vi "SwissSPAD2 Live.vi"() -> ()   [LabVIEW 2019]
uses:
  SS2 Live Internal Variables.ctl
  <vilib>/vision/Image Controls.llb/IMAQ Image.ctl
  SS2 Live_Image ROI Information.ctl
  Phasor/Image Binning Options.ctl
  SS2 Q [Element].ctl
  SS2 Q Event List.ctl
  Sound/System Sounds List.ctl
  SS2 Live_Settings List.ctl
  Image/Image Display to Clipboard Options.ctl
  Image/Image Display Palette Information.ctl
  Image/Image Display Palette Type.ctl
  SS2 Live_Internal Data List.ctl
  SS2 Live_Windows List.ctl
  SS2 Live_Globals.vi
  C:/UCLA Thinkpad Google Drive/LabVIEW 2019 SP1/builds/SS2 Live Distribution/Opal Kelly/C# Wrapper/libFrontPanel-csharp.dll
  Opal Kelly/C# Wrapper/libFrontPanel-csharp.dll
  Variant/Variant to Data/Variant to Data.lvlib
  Notebook/Notebook.lvlib
  Rich Text Box/Rich Text Box.lvlib
panel:
  out "Image":T1(plugin-control)
  out "Saving in progress":bool
  out "Progress":u8(slide) scale=0.0..100.0
  in  "Record":bool
  in  "Animated Busy Icon":bool=TRUE
  out "Message":string
  in  "Live":bool
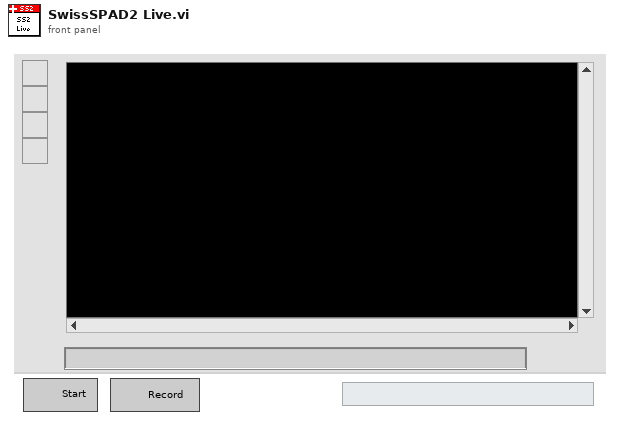
[diagram p1: front panel]
types:
  T1 = typedef "IMAQ Image.ctl" = refnum<image>
  T2 = typedef "SS2 Q [Element].ctl" = cluster{"SS2 Q Event":T3, "Data":variant}
  T3 = typedef "SS2 Q Event List.ctl" = enum16{"---- UI ----", "Idle", "Initialization", "Quit", "---- DAQ ----", "Start Recording", "Start Live Acquisition", "Initialize Recording Mode", "Initialize FPGA (Live Mode)", "Get Image Set", "Get Single Image", "Update Image Display", "Stop Live Acquisition", "Stop Data Recording", "---- Image ----", "Copy Data to Clipboard", "Set Image Palette", "Save Displayed Image with Overlay", "Save Image Data as TIFF"}
  T4 = typedef "SS2 Live Internal Variables.ctl" = cluster{"okCFrontPanelDevices Refnum":refnum<k24>, "Device Refnum":refnum<k24>, "Display Image":T1, "# Live Images":i32, "relative s":dbl, "# Image Sets":i32, "Message":string, "Current Image Set":i32, "# Datasets":i32, "Current Dataset":i32, "Live Mode":bool, "Recording Mode":bool, "Record Button":refnum<vi>, "Live Button":refnum<vi>, "SS2 Live Gate Data Q Name":string, "Discard First Image":bool, "Image Information":T5, "Image Binning Options":T6}
  T5 = typedef "SS2 Live_Image ROI Information.ctl" = cluster{"Save ROI Only":bool, "Left":u16, "Top":u16, "Right":u16, "Bottom":u16, "Use Current ROI":bool}
  T6 = typedef "Image Binning Options.ctl" = cluster{"Use Image Binning":bool, "X Bin":i32, "Y Bin":i32}
  T7 = typedef "SS2 Live_Settings List.ctl" = enum16{"FPGA:Bitfile Path", "FPGA:Bitfile Version", "Acquisition Parameters:SS2 DAQ Parameters", "Acquisition Parameters:Gate Configuration Array", "Acquisition Parameters:Buffer Size (# Gates)", "File Information:File Information", "File Information:# Datasets in Series", "Image Parameters:Image ROI Information", "Image Parameters:Image Binning Options", "UI Parameters:Histogram Bins Number"}
  T8 = typedef "System Sounds List.ctl" = enum16{"Alarm01", "Alarm02", "Alarm03", "Alarm04", "Alarm05", "Alarm06", "Alarm07", "Alarm08", "Alarm09", "Alarm10", "chimes", "chord", "ding", "notify", "recycle", "Ring01", "Ring02", "Ring03", "Ring04", "Ring05", "Ring06", "Ring07", "Ring08", "Ring09", "Ring10", "ringout", "Speech Off", "Speech On", "Speech Sleep", "tada", "Windows Background", "Windows Balloon", "Windows Battery Critical", "Windows Battery Low", "Windows Critical Stop", "Windows Default", "Windows Ding", "Windows Error", "Windows Exclamation", "Windows Feed Discovered", "Windows Foreground", "Windows Hardware Fail", "Windows Hardware Insert", "Windows Hardware Remove", "Windows Information Bar", "Windows Logoff Sound", "Windows Logon", "Windows Menu Command", "Windows Message Nudge", "Windows Minimize", "Windows Navigation Start", "Windows Notify Calendar", "Windows Notify Email", "Windows Notify Messaging", "Windows Notify System Generic", "Windows Notify", "Windows Pop-up Blocked", "Windows Print complete", "Windows Proximity Connection", "Windows Proximity Notification", "Windows Recycle", "Windows Restore", "Windows Ringin", "Windows Ringout", "Windows Shutdown", "Windows Startup", "Windows Unlock", "Windows User Account Control"}
  T9 = typedef "Image Display to Clipboard Options.ctl" = cluster{"Include Overlay (T)":bool, "Image Only (T)":bool}
  T10 = cluster{"CtlRef":refnum<vi>, "Image to Clipboard Options":T9}
  T11 = typedef "Image Display Palette Information.ctl" = cluster{"Palette Name [# Colors,int?,inv?]":string, "Palette Type":T12, "Palette Colors":u32[], "Interpolate?":bool}
  T12 = typedef "Image Display Palette Type.ctl" = u32
  T13 = typedef "Rich Text Box.lvlib/Text Formatting.ctl" = cluster{"Font":string, "Text Color":T14, "Text Background Color":T14, "Text Style":enum16{"Regular", "Bold", "Italic", "Underline", "Strikeout"}, "Font Size (Points)":dbl, "Text Alignment":i32}
  T14 = typedef "Rich Text Box.lvlib/Text Colors.ctl" = enum16{"Unchanged", "Black", "Blue", "Gray", "Green", "Red", "White"}
  T15 = typedef "Save File Format.ctl" = enum16{"PNG", "JPEG", "BMP"}
  T16 = typedef "SS2 Live_Internal Data List.ctl" = enum16{"Number of pending file saving tasks", "File Saving Tasks Information", "Current Image ROI Information"}
  T17 = typedef "SS2 Live_Windows List.ctl" = enum16{"Settings Window", "Notebook Window", "Histogram Window", "About Window", "SS2 Live Window"}
  T18 = cluster{"Global Rectangle":i32[], "Contours":cluster{"Contour Type":u32, "ROI Type":u32, "Points":i32[]}[]}
  T19 = typedef "SS2 Live_File Saving Task Information.ctl" = cluster{"File Path":string, "# Saved Images":i32, "# Images (Total)":i32, "File Size (Bytes)":i64}
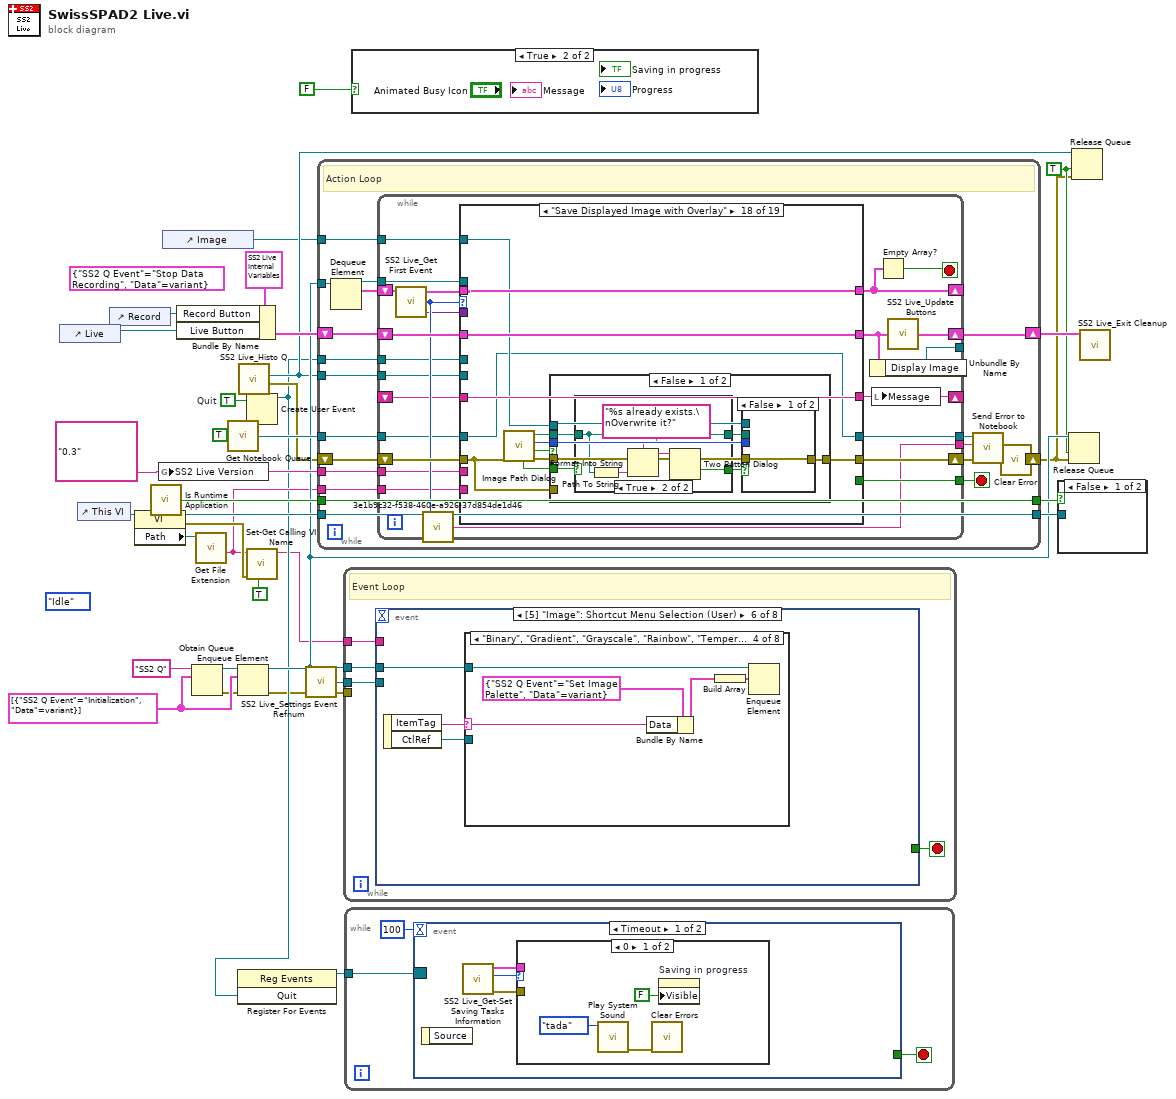
[diagram p0: block diagram]
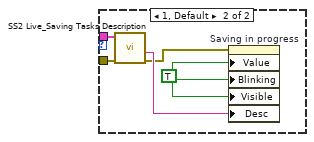
[diagram p2: hidden frame]
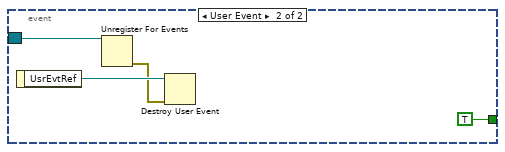
[diagram p3: hidden frame]
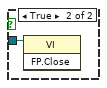
[diagram p5: hidden frame]
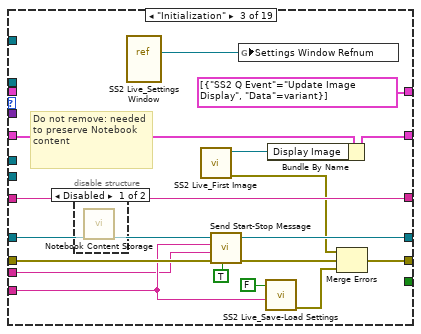
[diagram p8: hidden frame]
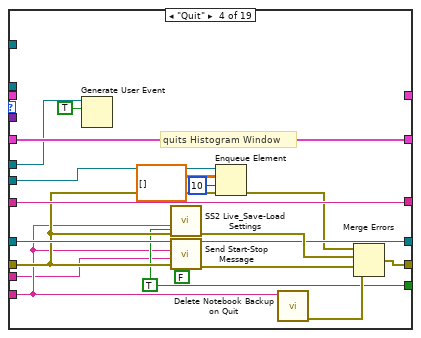
[diagram p10: hidden frame]
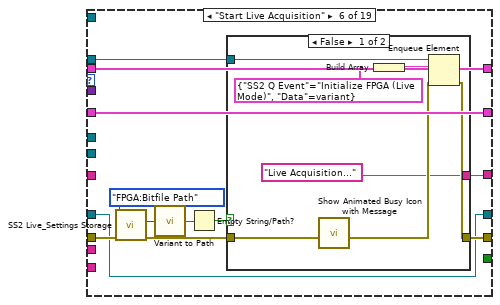
[diagram p12: hidden frame]
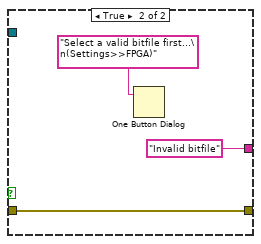
[diagram p13: hidden frame]
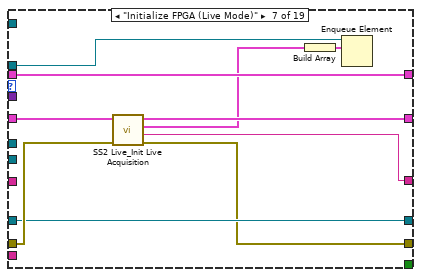
[diagram p14: hidden frame]
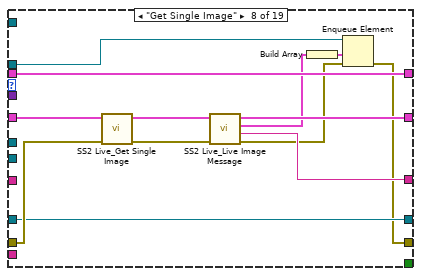
[diagram p15: hidden frame]
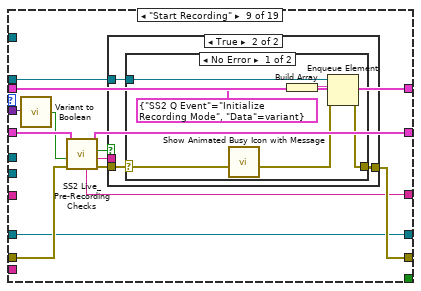
[diagram p16: hidden frame]
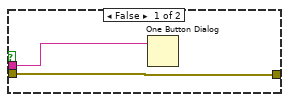
[diagram p17: hidden frame]
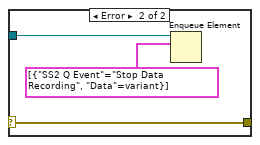
[diagram p18: hidden frame]
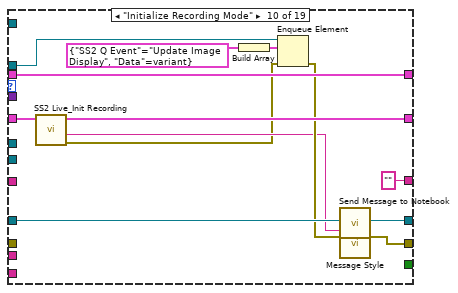
[diagram p19: hidden frame]
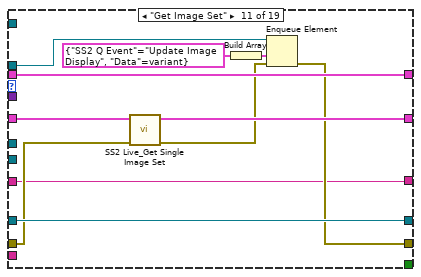
[diagram p20: hidden frame]
diagram:
  w9 = TRUE  # Quit
  (unwired) T2 {"SS2 Q Event"=enum."Stop Data Recording", "Data"=variant} ("f")
  w15 = TRUE ("force destroy? (F)")
  w18 = T2[] [{"SS2 Q Event"=enum."Initialization", "Data"=variant}] ("element")
  (unwired) SS2_Q_Event_List."Idle" ("SS2 Q Event")
  w20 = "0.3" ("SS2 Live Version")
  n1 = control-ref of="Live"() -> (w11:refnum<vi>)
  n2 = control-ref of="This VI"() -> (w32:refnum<vi>)
  n3 = control-ref of="Record"() -> (w10:refnum<vi>)
  n4 = property class="VI"(reference=w32) -> (reference out=w29:refnum<vi>, error out=w28:errorcluster, "Path"=w16:path)  [unwired: 1 in]
  n5 = call "Is Runtime Application.vi"() -> ("Runtime ?"=w34:bool)  [unwired: 8 in, 1 out]
  n6 = global write "SS2 Live_Globals.vi" "SS2 Live Version"(w20) -> ()
  n7 = control-ref of="Image"() -> (w1:refnum<vi>)
  n8 = Bundle By Name(cluster=T4 {"okCFrontPanelDevices Refnum"=refnum, "Device Refnum"=refnum, "Display Image"=refnum, "# Live Images"=0, "relative s"=nan, "# Image Sets"=0, "Message"="", "Current Image Set"=0, "# Datasets"=0, "Current Dataset"=0, "Live Mode"=FALSE, "Recording Mode"=FALSE, "Record Button"=refnum, "Live Button"=refnum, "SS2 Live Gate Data Q Name"="SS2 Live Gate Data Q", "Discard First Image"=FALSE, "Image Information"={"Save ROI Only"=FALSE, "Left"=0, "Top"=0, "Right"=0, "Bottom"=0, "Use Current ROI"=FALSE}, "Image Binning Options"={"Use Image Binning"=FALSE, "X Bin"=1, "Y Bin"=1}}, "Record Button"=w10, "Live Button"=w11) -> (w25:T4)
  n9 = Obtain Queue(name (unnamed)="SS2 Q", element data type=w18) -> (queue out=w21:refnum<queue>, error out=w5:errorcluster)  [unwired: 3 in, 1 out]
  n10 = call <vilib>:"Get File Extension.vi"("file"=w16) -> ("filename without extension"=w17:string)  [unwired: 6 in, 4 out]
  n11 = call "Get Notebook Queue.vi"("create if not found? (T)"=TRUE ("create if not found? (F)")) -> ("Notebook Queue"=w22:refnum<queue>)  [unwired: 8 in]
  n12 = Enqueue Element(queue=w21, element=w18, error in (no error)=w5) -> (queue out=w19:refnum<queue>, error out=w6:errorcluster)  [unwired: 1 in, 1 out]
  n13 = call "SS2 Live_Histo Q.vi"() -> ("error out"=w13:errorcluster, "SS2 Live Histo Q"=w12:refnum<queue>)  [unwired: 6 in]
  n14 = Create User Event(user event datatype=w9) -> (user event=w7:refnum<user-event>)  [unwired: 1 in, 1 out]
  n15 = register-events(w7) -> (reference out=w8:refnum<event-registration>)  [unwired: 2 in, 1 out]
  n16 = call "Set-Get Calling VI Name.vi"("Set/Get (F)"=TRUE, "Error In"=w28, "Calling VI Name"=w17) -> ("Calling VI Name"=w2:string)  [unwired: 7 in, 1 out]
  n17 = call "SS2 Live_Settings Event Refnum.vi"("Error In"=w6) -> ("Settings Event Refnum"=w3:refnum<user-event>, "Error Out"=w4:errorcluster)  [unwired: 7 in]
  n18 = while {
    tunnel: w19 -> [w55]
    tunnel: w34 -> [w50]
    tunnel: [w50] -> w33
    tunnel: w29 -> [w49]
    tunnel: [w49] -> w31
    shift-right: [w42] -> w14
    shift-left: w13 -> [w52]
    shift-right: [w47] -> w24
    shift-left: w25 -> [w48]
    tunnel: w22 -> [w46]
    tunnel: w20 -> [w40]
    tunnel: w17 -> [w39]
    tunnel: w12 -> [w38]
    tunnel: w7 -> [w37]
    tunnel: w1 -> [w36]
    stop <- w53 stop-if-true
    # "Action Loop"
    n19 = Dequeue Element(queue=w55) -> (queue out=w51:refnum<queue>, element=w54:T2[])  [unwired: 2 in, 2 out]
    n20 = while {
      tunnel: [w79] -> w53
      tunnel: w51 -> [w77]
      shift-right: [w76] -> w45
      shift-left: w52 -> [w78]
      shift-right: [w73] -> _
      shift-left: w54 -> [w75]
      shift-right: [w60] -> w47
      shift-left: w48 -> [w71]
      tunnel: w46 -> [w68]
      tunnel: [w65] -> w44
      tunnel: [w69] -> w41
      tunnel: w40 -> [w67]
      tunnel: w39 -> [w66]
      shift-right: [w64] -> _
      shift-left: _ -> [w63]
      tunnel: w38 -> [w61]
      tunnel: w37 -> [w59]
      tunnel: [w57] -> _
      tunnel: w36 -> [w56]
      stop <- w72 stop-if-true
      n21 = call "SS2 Live_Get First Event.vi"("SS2 Q Element"=w75) -> ("Data"=w62:variant, "SS2 Q Event"=w70:T3, "SS2 Q Elements"=w74:T2[])  [unwired: 2 in]
      n22 = call "3e1b9c32-f538-460e-a926-37d854de1d46.vi"("Enum"=w70) -> ("String"=w69:string)
      n23 = case shown="\"Save Displayed Image with Overlay\"" w70 {
        tunnel: [_ _ _ w113 _ _ _ _ _ _ _ _ _ _ _ _ _ _ _] -> w79
        tunnel: w78 -> [w84 w89 w98 w114 w128 w133 w157 w169 w182 _ w221 w228 w240 w257 w275 w283 w288 w305 w342]
        tunnel: w77 -> [_ _ _ _ _ w140 w160 w173 w186 w213 w224 w234 w246 w270 _ _ _ _ _]
        tunnel: [w84 w89 w104 w123 w128 w139 w151 w161 w185 w204 w215 w237 w244 w263 w275 w277 w289 w310 w342] -> w76
        tunnel: w74 -> [w83 w88 _ _ w127 w137 w158 w171 w184 w211 w223 w236 _ _ w274 w287 w302 w314 w341]
        tunnel: [w83 w88 T2[] [{"SS2 Q Event"=enum."Update Image Display", "Data"=variant}] ("SS2 Q Elements") _ w127 w137 w158 w171 w184 w211 w223 w236 _ _ w274 w287 w302 w314 w341] -> w73
        tunnel: w71 -> [w80 w87 w105 w121 w124 w136 w156 w170 w177 w208 w220 w232 w241 w251 w271 w282 w293 w313 w340]
        tunnel: [w80 w87 w92 w121 w124 w136 w154 w166 w176 w207 w217 w230 w239 w268 w271 w282 w293 w313 w340] -> w58
        tunnel: w61 -> [_ _ _ w117 _ _ _ _ _ _ _ _ _ _ _ _ _ _ _]
        tunnel: w68 -> [w82 w86 w100 w115 w126 w130 w155 w167 w181 w206 w222 w235 w243 w265 w273 w286 w301 w303 w339]
        tunnel: w67 -> [_ _ w96 w109 _ _ _ _ _ _ _ _ _ _ _ _ _ _ _]
        tunnel: w66 -> [_ _ w97 w110 _ _ _ _ _ _ _ _ _ _ _ _ _ _ _]
        tunnel: [w82 w86 w100 w115 w126 w130 w155 w167 w181 w206 w222 w235 w243 w265 w273 w286 w301 w303 w339] -> w65
        tunnel: [w81 w85 w102 w120 w125 w129 w152 w163 w179 "" ("Message") w214 w226 "Live Mode stopped" ("Message") w262 w272 w285 w300 w312 w338] -> w64
        tunnel: w63 -> [w81 w85 w102 w120 w125 _ _ _ _ _ w214 w225 _ _ w272 w285 w300 w312 w338]
        tunnel: w62 -> [_ _ _ _ _ _ _ _ w175 _ _ _ _ _ _ w284 w295 _ _]
        tunnel: w59 -> [_ _ _ w108 _ _ _ _ _ _ _ _ _ _ _ _ _ _ _]
        tunnel: w56 -> [_ _ _ _ _ _ _ _ _ _ _ _ _ _ _ _ w290 w311 _]
        frame "---- UI ----" {
        }
        frame "Idle", Default {
        }
        frame "Initialization" {
          # "Do not remove: needed to preserve Notebook content"
          n24 = disable-structure shown="Disabled" {
            frame Disabled {
              n25 = call "Notebook Content Storage.vi"() -> ()  [unwired: 10 in, 2 out]
            }
            frame Enabled {
            }
          }
          n26 = vi-ref "SS2 Live_Settings Window.vi"() -> (w101:refnum<vi>)
          n27 = call "SS2 Live_First Image.vi"() -> ("error out"=w90:errorcluster, "Image"=w91:T1)  [unwired: 10 in]
          n28 = call "Send Start-Stop Message.vi"("Start(T)/Stop(F)"=TRUE ("Start(F)/Stop(T)"), "Error In"=w98, "Version number"=w96, "Software Name"=w97, "Notebook Queue"=w100) -> ("Error Out"=w99:errorcluster)  [unwired: 6 in]
          n29 = global write "SS2 Live_Globals.vi" "Settings Window Refnum"(w101) -> ()
          n30 = call "SS2 Live_Save-Load Settings.vi"("Load(F)/Save (T)"=FALSE, "App Name"=w97) -> ("Error Out"=w103:errorcluster)  [unwired: 8 in, 1 out]
          n31 = Bundle By Name(cluster=w105, "Display Image"=w91) -> (w92:T4)
          n32 = Merge Errors(w90, w99, w103) -> (w104:errorcluster)
        }
        frame "Quit" {
          w113 = TRUE
          # "quits Histogram Window"
          n33 = Generate User Event(user event=w108, event data cluster=TRUE ("event data")) -> ()  [unwired: 2 in, 2 out]
          n34 = call "SS2 Live_Save-Load Settings.vi"("Load(F)/Save (T)"=w113, "Error In"=w114, "App Name"=w110) -> ("Error Out"=w122:errorcluster)  [unwired: 7 in, 1 out]
          n35 = call "Send Start-Stop Message.vi"("Start(T)/Stop(F)"=FALSE, "Error In"=w114, "Version number"=w109, "Software Name"=w110, "Notebook Queue"=w115) -> ("Error Out"=w111:errorcluster)  [unwired: 6 in]
          n36 = Enqueue Element(queue=w117, element=sgl[][] [], timeout in ms (-1)=10, error in (no error)=w114) -> (error out=w112:errorcluster)  [unwired: 2 out]
          n37 = call "Delete Notebook Backup on Quit.vi"("Main VI Name"=w110) -> ("Error Out"=w119:errorcluster)  [unwired: 10 in]
          n38 = Merge Errors(w112, w122, w111, w119) -> (w123:errorcluster)
        }
        frame "---- DAQ ----" {
        }
        frame "Start Live Acquisition" {
          n39 = call "SS2 Live_Settings Storage.vi"("Error In"=w133, "Settings List"=SS2_Live_Settings_List."FPGA:Bitfile Path") -> ("Error Out"=w134:errorcluster, "Variant Data out"=w132:variant)  [unwired: 8 in]
          n40 = call "Variant to Path.vi"("Variant"=w132) -> ("Path"=w131:path)  [unwired: 8 in]
          n41 = Empty String/Path?(string/path=w131) -> (empty?=w138:bool)
          n42 = case shown="False" w138 {
            tunnel: w140 -> [w145 _]
            tunnel: [w142 w150] -> w139
            tunnel: w134 -> [w146 w150]
            tunnel: ["Live Acquisition..." ("Message") "Invalid bitfile" ("Message")] -> w129
            frame False {
              n43 = call "Show Animated Busy Icon with Message.vi"("Error In"=w146) -> ("Error Out"=w143:errorcluster)  [unwired: 10 in]
              n44 = Build Array(T2 {"SS2 Q Event"=enum."Initialize FPGA (Live Mode)", "Data"=variant} ("SS2 Live Atomic Action")) -> (w144:T2[])
              n45 = Enqueue Element(queue=w145, element=w144, error in (no error)=w143) -> (error out=w142:errorcluster)  [unwired: 1 in, 2 out]
            }
            frame True {
              n46 = One Button Dialog(message="Select a valid bitfile first...\n(Settings>>FPGA)") -> ()  [unwired: 1 in, 1 out]
            }
          }
        }
        frame "Initialize FPGA (Live Mode)" {
          n47 = call "SS2 Live_Init Live Acquisition.vi"("error in (no error)"=w157, "SS2 Live Internal Variables in"=w156) -> ("error out"=w151:errorcluster, "Message"=w152:string, "SS2 Live Atomic Action"=w153:T2, "SS2 Live Internal Variables out"=w154:T4)  [unwired: 6 in]
          n48 = Build Array(w153) -> (w159:T2[])
          n49 = Enqueue Element(queue=w160, element=w159) -> ()  [unwired: 2 in, 3 out]
        }
        frame "Get Single Image" {
          n50 = call "SS2 Live_Get Single Image.vi"("error in (no error)"=w169, "SS2 Live Internal Variables"=w170) -> ("error out"=w165:errorcluster, "SS2 Live Internal Variables out"=w168:T4)  [unwired: 8 in]
          n51 = call "SS2 Live_Live Image Message.vi"("error in (no error)"=w165, "SS2 Live Internal Variables"=w168) -> ("error out"=w162:errorcluster, "Message"=w163:string, "SS2 Live Atomic Action"=w164:T2, "SS2 Live Internal Variables"=w166:T4)  [unwired: 6 in]
          n52 = Build Array(w164) -> (w172:T2[])
          n53 = Enqueue Element(queue=w173, element=w172, error in (no error)=w162) -> (error out=w161:errorcluster)  [unwired: 1 in, 2 out]
        }
        frame "Start Recording" {
          n54 = call "Variant to Boolean.vi"("Variant"=w175) -> ("Value"=w174:bool)  [unwired: 8 in]
          n55 = call "SS2 Live_Pre-Recording Checks.vi"("error in (no error)"=w182, "Init Series?"=w174, "SS2 Live Internal Variables in"=w177) -> ("error out"=w183:errorcluster, "Message"=w178:string, "Ready?"=w180:bool, "SS2 Live Internal Variables out"=w176:T4, "Verbose Message"=w179:string)  [unwired: 4 in]
          n56 = case shown="True" w180 {
            tunnel: w186 -> [_ w190]
            tunnel: [w188 w189] -> w185
            tunnel: w183 -> [w188 w191]
            tunnel: w178 -> [w187 _]
            frame False {
              n57 = One Button Dialog(message=w187) -> ()  [unwired: 1 in, 1 out]
            }
            frame True {
              n58 = case shown="No Error" w191 {
                selector: w191 -> [w196 w200]
                tunnel: w190 -> [w195 w199]
                tunnel: [w192 w200] -> w189
                frame No Error {
                  n59 = call "Show Animated Busy Icon with Message.vi"("Error In"=w196) -> ("Error Out"=w193:errorcluster)  [unwired: 10 in]
                  n60 = Build Array(T2 {"SS2 Q Event"=enum."Initialize Recording Mode", "Data"=variant} ("SS2 Live Atomic Action")) -> (w194:T2[])
                  n61 = Enqueue Element(queue=w195, element=w194, error in (no error)=w193) -> (error out=w192:errorcluster)  [unwired: 1 in, 2 out]
                }
                frame Error {
                  n62 = Enqueue Element(queue=w199, element=T2[] [{"SS2 Q Event"=enum."Stop Data Recording", "Data"=variant}]) -> ()  [unwired: 2 in, 3 out]
                }
              }
            }
          }
        }
        frame "Initialize Recording Mode" {
          n63 = call "SS2 Live_Init Recording.vi"("SS2 Live Internal Variables in"=w208) -> ("Error Out"=w201:errorcluster, "Notebook Message"=w203:string, "SS2 Live Internal Variables out"=w207:T4)  [unwired: 8 in]
          n64 = Build Array(T2 {"SS2 Q Event"=enum."Update Image Display", "Data"=variant} ("SS2 Live Queue Element Array")) -> (w212:T2[])
          n65 = Enqueue Element(queue=w213, element=w212, error in (no error)=w201) -> (error out=w205:errorcluster)  [unwired: 1 in, 2 out]
          n66 = call "Message Style.vi"() -> ("Message Formatting"=w202:T13)
          n67 = call "Send Message to Notebook.vi"("Notebook Queue"=w206, "Message"=w203, "Error In"=w205, "Text Formatting"=w202) -> ("Error Out"=w204:errorcluster)  [unwired: 15 in]
        }
        frame "Get Image Set" {
          n68 = call "SS2 Live_Get Single Image Set.vi"("error in (no error)"=w221, "SS2 Live Internal Variables"=w220) -> ("error out"=w216:errorcluster, "SS2 Live Internal Variables out"=w217:T4)  [unwired: 8 in]
          n69 = Build Array(T2 {"SS2 Q Event"=enum."Update Image Display", "Data"=variant} ("SS2 Live Atomic Action")) -> (w219:T2[])
          n70 = Enqueue Element(queue=w224, element=w219, error in (no error)=w216) -> (error out=w215:errorcluster)  [unwired: 1 in, 2 out]
        }
        frame "Update Image Display" {
          n71 = Unbundle By Name(w232) -> ("Display Image"=→"Image":T1)
          n72 = call "SS2 Live_Next Image Acquisition Step.vi"("Error In"=w228, "Message in"=w225, "SS2 Live Internal Variables in"=w232) -> ("Error Out"=w227:errorcluster, "Message out"=w226:string, "SS2 Live Atomic Action"=w229:T2, "SS2 Live Internal Variables out"=w230:T4)  [unwired: 5 in]
          n73 = Build Array(w229) -> (w233:T2[])
          n74 = Enqueue Element(queue=w234, element=w233, error in (no error)=w227) -> (error out=w237:errorcluster)  [unwired: 1 in, 2 out]
        }
        frame "Stop Live Acquisition" {
          w238 = FALSE ("Record")
          n75 = Flush Queue(queue=w246, error in (no error)=w240) -> (error out=w245:errorcluster)  [unwired: 2 out]
          n76 = call "Hide Animated Busy Icon with Message.vi"("Error In"=w245) -> ("Error Out"=w244:errorcluster)  [unwired: 10 in]
          n77 = property on="Live" class="Bool (strict)"("Value"=w238) -> ()  [unwired: 2 in, 2 out]
          n78 = Bundle By Name(cluster=w241, "Live Mode"=w238) -> (w239:T4)
        }
        frame "Stop Data Recording" {
          w252 = FALSE ("Record")
          w262 = "Data Recording stopped" ("Message")
          # "Stops data saving"
          n79 = Flush Queue(queue=w270) -> (error out=w269:errorcluster)  [unwired: 1 in, 2 out]
          n80 = call "Current Date & Time String.vi"("Error In"=w257) -> ("Error Out"=w258:errorcluster, "time string"=w259:string, "date string"=w260:string)  [unwired: 8 in]
          n81 = call "Hide Animated Busy Icon with Message.vi"("Error In"=w269) -> ("Error Out"=w264:errorcluster)  [unwired: 10 in]
          n82 = Unbundle By Name(w251) -> ("SS2 Live Gate Data Q Name"=w250:string)
          n83 = Format Into String(format string=" on %s at %s", initial string=w262, error in=w258, w260, w259) -> (resulting string=w254:string, error out=w255:errorcluster)
          n84 = property on="Record" class="Bool (strict)"("Value"=w252) -> ()  [unwired: 2 in, 2 out]
          n85 = call "Play System Sound.vi"("Windows Sound"=System_Sounds_List."notify") -> ("Error Out"=w247:errorcluster)  [unwired: 10 in]
          n86 = call <vilib>:"Clear Errors.vi"("error in (no error)"=w247) -> ()  [unwired: 5 in, 2 out]
          n87 = Merge Errors(w264, w255) -> (w256:errorcluster)
          n88 = call "SS2 Live_Gate Data Q.vi"("SS2 Live Gate Data Q Name"=w250) -> ("SS2 Live Gate Data Q"=w249:refnum<queue>)  [unwired: 5 in, 1 out]
          n89 = Bundle By Name(cluster=w251, "Current Image Set"=2147483647, "Recording Mode"=w252) -> (w268:T4)
          n90 = call "Message Style.vi"() -> ("Message Formatting"=w253:T13)
          n91 = call "Send Message to Notebook.vi"("Notebook Queue"=w265, "Message"=w254, "Error In"=w256, "Text Formatting"=w253) -> ("Error Out"=w263:errorcluster)  [unwired: 15 in]
          n92 = Enqueue Element(queue=w249, element=u8[][] [] ("second subarray")) -> ()  [unwired: 2 in, 3 out]
        }
        frame "---- Image ----" {
        }
        frame "Copy Data to Clipboard" {
          n93 = Variant To Data(error in=w283, type=T10 {"CtlRef"=refnum, "Image to Clipboard Options"={"Include Overlay (T)"=FALSE, "Image Only (T)"=FALSE}} ("output cluster"), Variant=w284) -> (data=w280:T10, error out=w278:errorcluster)
          n94 = Unbundle(w280) -> ("CtlRef"=w279:refnum<vi>, "Image to Clipboard Options"=w276:T9)
          n95 = call "Image Display_Copy Image to Clipboard.vi"("Error In"=w278, "Image to Clipboard Options"=w276, "Display Image Control Refnum"=w279) -> ("Error Out"=w277:errorcluster)  [unwired: 8 in]
        }
        frame "Set Image Palette" {
          n96 = call "Variant to String.vi"("Variant"=w295) -> ("String"=w294:string)  [unwired: 8 in]
          n97 = call "Get User Palette Choice.vi"("Error In"=w288, "Palette"=w294) -> ("Error Out"=w292:errorcluster, "Palette Colors"=w298:u32[], "Palette Type"=w299:T12, "Palette Name (# Colors)"=w296:string)  [unwired: 3 in, 3 out]
          n98 = Bundle(cluster=T11 {"Palette Name [# Colors,int?,inv?]"="", "Palette Type"=0, "Palette Colors"=[], "Interpolate?"=FALSE} ("Image Display Palette Information"), "Palette Name [# Colors,int?,inv?]"=w296, "Palette Type"=w299, "Palette Colors"=w298) -> (w291:T11)  [unwired: 1 in]
          n99 = call "Image Display_Set Colot Palette.vi"("Error In"=w292, "Image Display Palette Information"=w291, "Display Image Control Refnum"=w290) -> ("Error Out"=w289:errorcluster)  [unwired: 8 in]
        }
        frame "Save Displayed Image with Overlay" {
          n100 = call "Image Path Dialog.vi"("error in (no error)"=w305) -> ("error out"=w308:errorcluster, "Cancelled?"=w306:bool, "Saved Image File Format"=w307:T15, "Selected Path"=w309:path, "Exists?"=w304:bool)  [unwired: 6 in]
          n101 = case shown="False" w306 {
            tunnel: w311 -> [w322 _]
            tunnel: [w321 w337] -> w310
            tunnel: w309 -> [w317 _]
            tunnel: w308 -> [w320 _]
            tunnel: w307 -> [w319 _]
            tunnel: w305 -> [_ w337]
            tunnel: w304 -> [w318 _]
            frame False {
              n102 = case shown="True" w318 {
                selector: w318 -> [w330 _]
                tunnel: w317 -> [w331 w332]
                tunnel: [w331 w332] -> w316
                tunnel: [w329 w336] -> w315
                frame False {
                  n103 = Not(x=w330) -> (.not. x?=w329:bool)
                }
                frame True {
                  n104 = Path To String(path=w332) -> (string=w334:string)
                  n105 = Format Into String(format string="%s already exists.\nOverwrite it?", w334) -> (resulting string=w333:string)  [unwired: 2 in, 1 out]
                  n106 = Two Button Dialog(message=w333) -> (T button?=w336:bool)  [unwired: 2 in]
                }
              }
              n107 = case shown="False" w315 {
                tunnel: w322 -> [_ w328]
                tunnel: [w323 w327] -> w321
                tunnel: w320 -> [w323 w326]
                tunnel: w319 -> [_ w325]
                tunnel: w316 -> [_ w324]
                frame False {
                }
                frame True {
                  n108 = call "Save Displayed Image.vi"("error in (no error)"=w326, "Saved Image File Format"=w325, "File Path in"=w324, "Display Image Control Refnum"=w328) -> ("Error Out"=w327:errorcluster)  [unwired: 6 in, 1 out]
                }
              }
            }
            frame True {
            }
          }
        }
        frame "Save Image Data as TIFF" {
          # "#TODO"
        }
      }
      n109 = Unbundle By Name(w58) -> ("Display Image"=w57:T1)
      n110 = local write "Message"(w64) -> ()
      n111 = Empty Array?(array=w73) -> (empty?=w72:bool)
      n112 = call "SS2 Live_Update Buttons.vi"("SS2 Live Internal Variables in"=w58) -> ("SS2 Live Internal Variables out"=w60:T4)  [unwired: 6 in]
    }
    n113 = call "Send Error to Notebook.vi"("error in (no error)"=w45, "State Machine Case Error Source"=w41, "Notebook Q"=w44) -> ("Error Out"=w43:errorcluster)  [unwired: 8 in]
    n114 = call "Clear Error.vi"("Error In"=w43) -> ("no Error Out"=w42:errorcluster)  [unwired: 8 in]
  }
  n115 = while {
    tunnel: w19 -> [w345]
    tunnel: w4 -> [_]
    tunnel: w3 -> [w344]
    tunnel: w2 -> [w343]
    stop <- w346 stop-if-true
    # "Event Loop"
    n116 = event shown="[5] \"Image\": Shortcut Menu Selection (User)" {
      selector: _ -> [_ _ _ _ _ _ _ _]
      dyn-events: _ -> [_ _ _ _ _ _ _ _]
      timeout: _ -> [_ _ _ _ _ _ _ _]
      tunnel: [w351 w357 _ _ TRUE _ _ _] -> w346
      tunnel: w345 -> [w355 w358 w385 w401 w424 w425 _ _]
      tunnel: w344 -> [_ _ _ _ _ _ _ w460]
      tunnel: w343 -> [_ _ _ _ _ _ _ w459]
      event Panel Close? {
        n117 = event-data() -> ()  [unwired: 1 in, 1 out]
        n118 = local read "Record"() -> (w353:bool)
        n119 = call "SS2 Live_Internal Data Storage.vi"("SS2 Live Data"=SS2_Live_Internal_Data_List."Number of pending file saving tasks") -> ("Variant"=w348:variant)  [unwired: 8 in, 2 out]
        n120 = local read "Live"() -> (w354:bool)
        n121 = call "Variant to I32.vi"("Variant"=w348) -> ("Value"=w347:i32)  [unwired: 8 in]
        n122 = Not Equal To 0?(x=w347) -> (x != 0?=w352:bool)
        n123 = Build Array(w354, w353, w352) -> (w350:bool[])
        n124 = call "SS2 Live_Ready to Quit.vi"("Flags"=w350, "SS2 Live Queue in"=w355) -> ("Ready to Quit?"=w351:bool)  [unwired: 8 in, 1 out]
        n125 = event-data("Discard?"=TRUE) -> ()  [unwired: 1 in, 1 out]
      }
      event Menu Selection (User) {
        n126 = event-data() -> ("ItemTag"=w359:string)  [unwired: 1 in]
        n127 = case shown="\"Quit\"" w359 {
          tunnel: w358 -> [_ _ w366 _ _ _ _ _]
          tunnel: [_ _ w365 _ _ _ _ _] -> w357
          frame "", Default {
          }
          frame "------ File -------" {
          }
          frame "Quit" {
            n128 = local read "Record"() -> (w368:bool)
            n129 = local read "Live"() -> (w367:bool)
            n130 = call "SS2 Live_Internal Data Storage.vi"("SS2 Live Data"=SS2_Live_Internal_Data_List."Number of pending file saving tasks") -> ("Variant"=w361:variant)  [unwired: 8 in, 2 out]
            n131 = call "Variant to I32.vi"("Variant"=w361) -> ("Value"=w360:i32)  [unwired: 8 in]
            n132 = Not Equal To 0?(x=w360) -> (x != 0?=w363:bool)
            n133 = Build Array(w367, w368, w363) -> (w364:bool[])
            n134 = call "SS2 Live_Ready to Quit.vi"("Flags"=w364, "SS2 Live Queue in"=w366) -> ("Ready to Quit?"=w365:bool)  [unwired: 8 in, 1 out]
          }
          frame "----- Windows -------" {
          }
          frame "Settings" {
            n135 = call "SS2 Live_Get Ancillary Window Path.vi"("SS2 Live Windows"=SS2_Live_Windows_List."Settings Window") -> ("Error Out"=w369:errorcluster, "VI Path"=w370:path)  [unwired: 9 in]
            n136 = call "Run Vi.vi"("VI Path"=w370, "error in (no error)"=w369) -> ()  [unwired: 6 in, 2 out]
          }
          frame "Histogram" {
            n137 = call "SS2 Live_Get Ancillary Window Path.vi"("SS2 Live Windows"=SS2_Live_Windows_List."Histogram Window") -> ("Error Out"=w372:errorcluster, "VI Path"=w373:path)  [unwired: 9 in]
            n138 = call "Run Vi.vi"("VI Path"=w373, "error in (no error)"=w372) -> ()  [unwired: 6 in, 2 out]
          }
          frame "Notebook" {
            n139 = call "SS2 Live_Get Ancillary Window Path.vi"("SS2 Live Windows"=SS2_Live_Windows_List."Notebook Window") -> ("Error Out"=w376:errorcluster, "VI Path"=w377:path)  [unwired: 9 in]
            n140 = call "Run Vi.vi"("VI Path"=w377, "error in (no error)"=w376, "Start Hidden? (F)"=TRUE) -> ()  [unwired: 5 in, 2 out]
          }
          frame "About" {
            n141 = call "SS2 Live_Get Ancillary Window Path.vi"("SS2 Live Windows"=SS2_Live_Windows_List."About Window") -> ("Error Out"=w379:errorcluster, "VI Path"=w380:path)  [unwired: 9 in]
            n142 = call "Run Vi.vi"("VI Path"=w380, "error in (no error)"=w379) -> ()  [unwired: 6 in, 2 out]
          }
        }
      }
      event "Live": Value Change {
        n143 = event-data() -> ("OldVal"=w382:bool)  [unwired: 1 in]
        n144 = local read "Record"() -> (w383:bool)
        n145 = case shown="False" w383 {
          tunnel: w385 -> [w387 _]
          tunnel: "Live" -> [w386 _]
          tunnel: w382 -> [_ w396]
          frame False {
            n146 = case shown="True" w386 {
              tunnel: w387 -> [w392 w395]
              frame False {
                n147 = Flush Queue(queue=w392) -> (queue out=w390:refnum<queue>, error out=w389:errorcluster)  [unwired: 1 in, 1 out]
                n148 = Build Array(T2 {"SS2 Q Event"=enum."Stop Live Acquisition", "Data"=variant} ("element")) -> (w391:T2[])
                n149 = Enqueue Element At Opposite End(queue=w390, element=w391, error in (no error)=w389) -> ()  [unwired: 1 in, 3 out]
              }
              frame True {
                n150 = Build Array(T2 {"SS2 Q Event"=enum."Start Live Acquisition", "Data"=variant} ("element")) -> (w393:T2[])
                n151 = Enqueue Element(queue=w395, element=w393) -> ()  [unwired: 2 in, 3 out]
              }
            }
          }
          frame True {
            n152 = property on="Live" class="Bool (strict)"("Value"=w396) -> ()  [unwired: 2 in, 2 out]
            n153 = One Button Dialog(message="Recording in progress: wait or abort before switching to Live Mode") -> ()  [unwired: 1 in, 1 out]
          }
        }
      }
      event "Record": Value Change {
        n154 = event-data() -> ("OldVal"=w398:bool)  [unwired: 1 in]
        n155 = local read "Live"() -> (w399:bool)
        n156 = case shown="False" w399 {
          tunnel: w401 -> [w403 _]
          tunnel: "Record" -> [w402 _]
          tunnel: w398 -> [_ w414]
          frame False {
            n157 = case shown="True" w402 {
              selector: w402 -> [_ w409]
              tunnel: w403 -> [w408 w413]
              frame False {
                n158 = Flush Queue(queue=w408) -> (queue out=w406:refnum<queue>, error out=w405:errorcluster)  [unwired: 1 in, 1 out]
                n159 = Build Array(T2 {"SS2 Q Event"=enum."Stop Data Recording", "Data"=variant} ("element")) -> (w407:T2[])
                n160 = Enqueue Element At Opposite End(queue=w406, element=w407, error in (no error)=w405) -> ()  [unwired: 1 in, 3 out]
              }
              frame True {
                n161 = Bundle By Name(cluster=T2 {"SS2 Q Event"=enum."Start Recording", "Data"=variant} ("element"), "Data"=w409) -> (w410:T2)
                n162 = Build Array(w410) -> (w411:T2[])
                n163 = Enqueue Element(queue=w413, element=w411) -> ()  [unwired: 2 in, 3 out]
              }
            }
          }
          frame True {
            n164 = property on="Record" class="Bool (strict)"("Value"=w414) -> ()  [unwired: 2 in, 2 out]
            n165 = One Button Dialog(message="Live mode on: Stop before switching to Recording Mode") -> ()  [unwired: 1 in, 1 out]
          }
        }
      }
      event Application Instance Close {
        n166 = event-data() -> ()  [unwired: 1 in, 1 out]
        n167 = Flush Queue(queue=w424) -> (queue out=w420:refnum<queue>)  [unwired: 1 in, 2 out]
        n168 = local read "Live"() -> (w419:bool)
        n169 = Select(t=T2 {"SS2 Q Event"=enum."Stop Live Acquisition", "Data"=variant} ("element"), s=w419, f=T2 {"SS2 Q Event"=enum."Stop Data Recording", "Data"=variant} ("element")) -> (s? t:f=w416:T2)
        n170 = Build Array(w416, T2 {"SS2 Q Event"=enum."Quit", "Data"=variant} ("element")) -> (w421:T2[])
        n171 = Enqueue Element(queue=w420, element=w421) -> ()  [unwired: 2 in, 3 out]
      }
      event "Image": Shortcut Menu Selection (User) {
        n172 = event-data() -> ("ItemTag"=w427:string, "CtlRef"=w426:refnum<vi>)  [unwired: 1 in]
        n173 = case shown="\"Binary\", \"Gradient\", \"Grayscale\", \"Rainbow\", \"Temperature\"" w427 {
          selector: w427 -> [_ _ _ w442 _ _ _ _]
          tunnel: w426 -> [_ w430 w437 _ _ _ w454 w456]
          tunnel: w425 -> [_ w434 w441 w446 w449 w452 _ _]
          frame "", Default {
          }
          frame "Copy Data to Clipboard" {
            n174 = Bundle("CtlRef"=w430, "Image to Clipboard Options"=T9 {"Include Overlay (T)"=TRUE, "Image Only (T)"=FALSE}) -> (w428:T10)  [unwired: 1 in]
            n175 = Bundle By Name(cluster=T2 {"SS2 Q Event"=enum."Copy Data to Clipboard", "Data"=variant} ("SS2 Q Element"), "Data"=w428) -> (w432:T2)
            n176 = Build Array(w432) -> (w431:T2[])
            n177 = Enqueue Element(queue=w434, element=w431) -> ()  [unwired: 2 in, 3 out]
          }
          frame "Copy Image Only (with Overlay)" {
            n178 = Bundle("CtlRef"=w437, "Image to Clipboard Options"=T9 {"Include Overlay (T)"=TRUE, "Image Only (T)"=TRUE}) -> (w435:T10)  [unwired: 1 in]
            n179 = Bundle By Name(cluster=T2 {"SS2 Q Event"=enum."Copy Data to Clipboard", "Data"=variant} ("SS2 Q Element"), "Data"=w435) -> (w439:T2)
            n180 = Build Array(w439) -> (w438:T2[])
            n181 = Enqueue Element(queue=w441, element=w438) -> ()  [unwired: 2 in, 3 out]
          }
          frame "Binary", "Gradient", "Grayscale", "Rainbow", "Temperature" {
            n182 = Bundle By Name(cluster=T2 {"SS2 Q Event"=enum."Set Image Palette", "Data"=variant} ("SS2 Q Element"), "Data"=w442) -> (w444:T2)
            n183 = Build Array(w444) -> (w443:T2[])
            n184 = Enqueue Element(queue=w446, element=w443) -> ()  [unwired: 2 in, 3 out]
          }
          frame "Save Displayed Image with Overlay" {
            n185 = Build Array(T2 {"SS2 Q Event"=enum."Save Displayed Image with Overlay", "Data"=variant} ("SS2 Q Element")) -> (w448:T2[])
            n186 = Enqueue Element(queue=w449, element=w448) -> ()  [unwired: 2 in, 3 out]
          }
          frame "Save Image Data as TIFF" {
            n187 = Build Array(T2 {"SS2 Q Event"=enum."Save Image Data as TIFF", "Data"=variant} ("SS2 Q Element")) -> (w451:T2[])
            n188 = Enqueue Element(queue=w452, element=w451) -> ()  [unwired: 2 in, 3 out]
          }
          frame "Zoom to Fit" {
            n189 = call "Image Display_Zoom to Fit.vi"("Keep Aspect Ratio (T)"=FALSE, "Display Image Control Refnum"=w454) -> ()  [unwired: 9 in, 1 out]
          }
          frame "Zoom to Fit (Keep Aspect Ratio)" {
            n190 = call "Image Display_Zoom to Fit.vi"("Keep Aspect Ratio (T)"=TRUE, "Display Image Control Refnum"=w456) -> ()  [unwired: 9 in, 1 out]
          }
        }
      }
      event "Saving in progress": Shortcut Menu Selection (User) {
        n191 = event-data() -> ("ItemTag"=w457:string)  [unwired: 1 in]
        n192 = case shown="\"Abort All Saving Tasks\"" w457 {
          frame "", Default {
          }
          frame "Abort All Saving Tasks" {
            n193 = call "SS2 Live_Abort Saving Tasks.vi"() -> ()  [unwired: 12 in]
          }
        }
      }
      event "Image": Mouse Up {
        n194 = event-data() -> ("CtlRef"=w465:refnum<vi>)  [unwired: 1 in]
        n195 = property class="ImageControl"(reference=w465) -> (error out=w463:errorcluster, "ROI"=w464:T18)  [unwired: 1 in, 1 out]
        n196 = call "SS2 Live_Internal Data Storage.vi"("Get(F)/Set"=TRUE, "SS2 Live Data"=SS2_Live_Internal_Data_List."Current Image ROI Information", "Error In"=w463, "Variant"=w464) -> ("Error Out"=w458:errorcluster)  [unwired: 5 in, 2 out]
        n197 = call "SS2 Live_Update Image Information Event.vi"("error in (no error)"=w458, "Calling VI Name"=w459, "User Event in"=w460) -> ()  [unwired: 9 in]
      }
    }
  }
  n198 = while {
    tunnel: w8 -> [w467]
    stop <- w466 stop-if-true
    n199 = event shown="[0] Timeout" {
      selector: w467 -> [_ w481]
      dyn-events: _ -> [_ _]
      timeout: 100 -> [_ _]
      tunnel: [_ TRUE] -> w466
      event Timeout {
        n200 = event-data() -> ()  [unwired: 1 in, 1 out]
        n201 = call "SS2 Live_Get-Set Saving Tasks Information.vi"() -> ("error out"=w469:errorcluster, "# Saving Tasks"=w471:i32, "Array of Saving Tasks Information"=w470:T19[])  [unwired: 8 in, 1 out]
        n202 = case shown="0" w471 {
          tunnel: w470 -> [_ w479]
          tunnel: w469 -> [_ w475]
          frame 0 {
            n203 = call "Play System Sound.vi"("Windows Sound"=System_Sounds_List."tada") -> ("Error Out"=w472:errorcluster)  [unwired: 10 in]
            n204 = call <vilib>:"Clear Errors.vi"("error in (no error)"=w472) -> ()  [unwired: 5 in, 2 out]
            n205 = property on="Saving in progress" class="Bool (strict)"("Visible"=FALSE) -> ()  [unwired: 2 in, 2 out]
          }
          frame 1, Default {
            w477 = TRUE ("Saving in progress")
            n206 = call "SS2 Live_Saving Tasks Description.vi"("Error In"=w475, "Array of Saving Tasks Information"=w479) -> ("Error Out"=w476:errorcluster, "Description"=w478:string)  [unwired: 8 in]
            n207 = property on="Saving in progress" class="Bool (strict)"(error in=w476, "Value"=w477, "Blinking"=w477, "Visible"=w477, "Desc"=w478) -> ()  [unwired: 1 in, 2 out]
          }
        }
      }
      event User Event {
        n208 = event-data() -> ("UsrEvtRef"=w483:refnum<user-event>)  [unwired: 1 in]
        n209 = Unregister For Events(event registration refnum=w481) -> (error out=w480:errorcluster)  [unwired: 1 in]
        n210 = Destroy User Event(user event=w483, error in=w480) -> ()  [unwired: 1 out]
      }
    }
  }
  n211 = case shown="True" FALSE {
    frame False {
    }
    frame True {
    }
  }
  n212 = case shown="False" w33 {
    tunnel: w31 -> [_ w484]
    frame False {
    }
    frame True {
      n213 = invoke class="VI" method="FP.Close"(reference=w484) -> ()  [unwired: 2 in, 3 out]
    }
  }
  n214 = Release Queue(queue=w19, force destroy? (F)=w15, error in (no error)=w14) -> ()  [unwired: 3 out]
  n215 = Release Queue(queue=w12, force destroy? (F)=w15, error in (no error)=w14) -> ()  [unwired: 3 out]
  n216 = call "SS2 Live_Exit Cleanup.vi"("SS2 Live Internal Variables"=w24) -> ()  [unwired: 11 in]
